vi "GoT (SubVI).vi"(0 "Error In 3":errorcluster, 1 "Error In 9":errorcluster, 5 "error in (no error)":errorcluster) -> (6 "Selected Octave 3":i32[](array[numeric]), 8 "Number_of_elements 9":dbl, 9 "Array 2":i32[](array[numeric]), 10 "Number_of_elements 3":dbl, 11 "Notes 2":i32[](array[numeric]), 12 "Status 3":i32[](array[numeric]), 13 "Time 2":dbl[](array[numeric]), 14 "Array 3":dbl[](array[numeric]), 15 "Error Out 3":errorcluster, 16 "Array":i32[](array[numeric]), 17 "Error Out 9":errorcluster, 18 "Number_of_elements 4":dbl, 19 "error out":errorcluster)   [LabVIEW 2016]
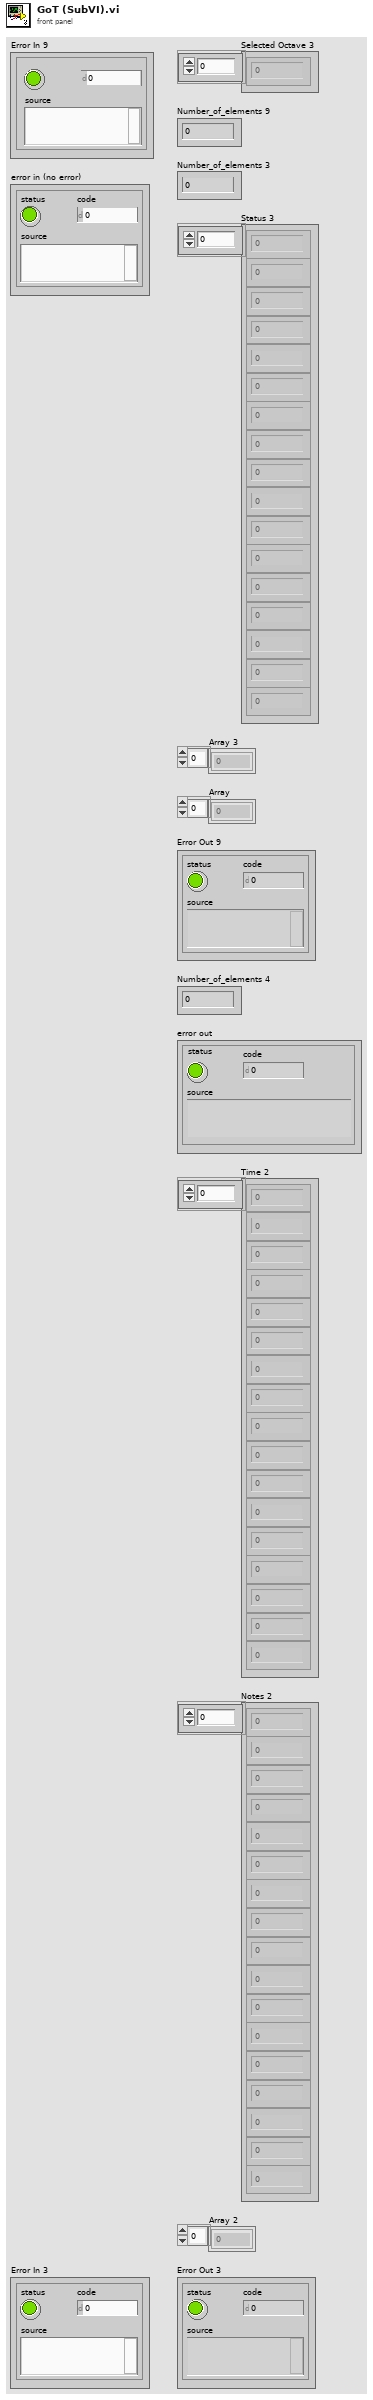
[diagram p1: front panel]
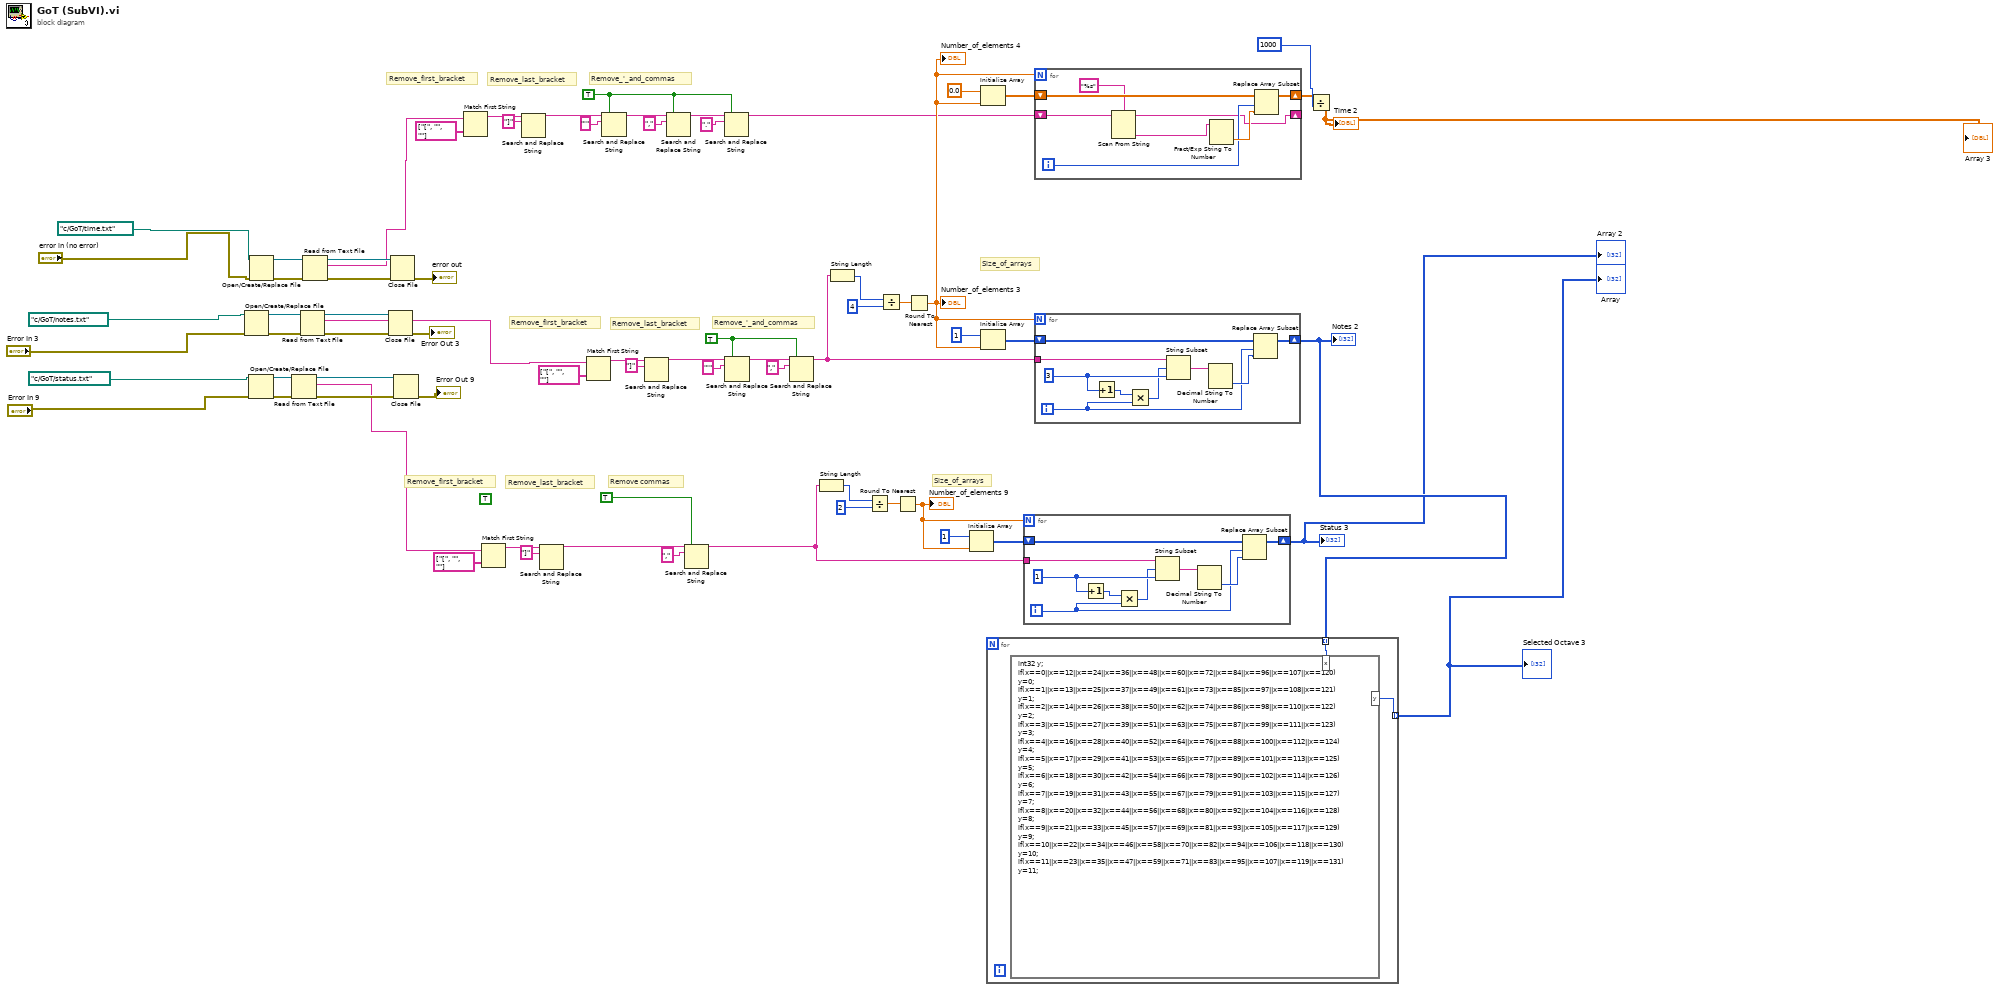
[diagram p0: block diagram]
diagram:
  (unwired) TRUE ("replace all? (F)")
  w13 = TRUE ("replace all? (F)")
  w27 = TRUE ("replace all? (F)")
  # "Size_of_arrays"
  # "Remove commas"
  # "Remove_last_bracket"
  # "Remove_first_bracket"
  # "Remove_'_and_commas"
  # "Remove_last_bracket"
  # "Remove_first_bracket"
  # "Size_of_arrays"
  # "Remove_'_and_commas"
  # "Remove_last_bracket"
  # "Remove_first_bracket"
  n1 = Open/Create/Replace File(file path (use dialog)=path "c:/GoT/notes.txt", error in="Error In 3") -> (refnum out=w65:refnum<file>, error out=w66:errorcluster)  [unwired: 4 in, 1 out]
  n2 = Open/Create/Replace File(file path (use dialog)=path "c:/GoT/status.txt", error in="Error In 9") -> (refnum out=w68:refnum<file>, error out=w67:errorcluster)  [unwired: 4 in, 1 out]
  n3 = Open/Create/Replace File(file path (use dialog)=path "c:/GoT/time.txt", error in="error in (no error)") -> (refnum out=w58:refnum<file>, error out=w57:errorcluster)  [unwired: 4 in, 1 out]
  n4 = Read from Text File(file (use dialog)=w68, error in=w67) -> (refnum out=w70:refnum<file>, text=w52:string, error out=w69:errorcluster)  [unwired: 2 in, 1 out]
  n5 = Read from Text File(file (use dialog)=w65, error in=w66) -> (refnum out=w62:refnum<file>, text=w33:string, error out=w63:errorcluster)  [unwired: 2 in, 1 out]
  n6 = Read from Text File(file (use dialog)=w58, error in=w57) -> (refnum out=w61:refnum<file>, text=w31:string, error out=w60:errorcluster)  [unwired: 2 in, 1 out]
  n7 = Close File(refnum=w62, error in=w63) -> (error out=→"Error Out 3":errorcluster)  [unwired: 1 out]
  n8 = Close File(refnum=w61, error in=w60) -> (error out=→"error out":errorcluster)  [unwired: 1 out]
  n9 = Close File(refnum=w70, error in=w69) -> (error out=→"Error Out 9":errorcluster)  [unwired: 1 out]
  n10 = Match First String(2:string[] ["[", "", ""] ("string array"), 3:w31) -> (1:w2:string)  [unwired: 1 out]
  n11 = Match First String(2:string[] ["[", "", ""] ("string array"), 3:w52) -> (1:w40:string)  [unwired: 1 out]
  n12 = Search and Replace String(input string=w2, search string="]") -> (result string=w4:string)  [unwired: 6 in, 3 out]
  n13 = Search and Replace String(input string=w40, search string="]") -> (result string=w42:string)  [unwired: 6 in, 3 out]
  n14 = Match First String(2:string[] ["[", "", ""] ("string array"), 3:w33) -> (1:w22:string)  [unwired: 1 out]
  n15 = Search and Replace String(replace all?=w27, input string=w4, search string="'") -> (result string=w7:string)  [unwired: 5 in, 3 out]
  n16 = Search and Replace String(input string=w22, search string="]") -> (result string=w20:string)  [unwired: 6 in, 3 out]
  n17 = Search and Replace String(replace all?=w27, input string=w7, search string=",") -> (result string=w24:string)  [unwired: 5 in, 3 out]
  n18 = Search and Replace String(replace all?=TRUE ("replace all? (F)"), input string=w42, search string=",") -> (result string=w49:string)  [unwired: 5 in, 3 out]
  n19 = Search and Replace String(replace all?=w27, input string=w24, search string=".") -> (result string=w25:string)  [unwired: 5 in, 3 out]
  n20 = Search and Replace String(replace all?=w13, input string=w20, search string="'") -> (result string=w17:string)  [unwired: 5 in, 3 out]
  n21 = Search and Replace String(replace all?=w13, input string=w17, search string=",") -> (result string=w12:string)  [unwired: 5 in, 3 out]
  n22 = String Length(string=w49) -> (length=w47:i32)
  n23 = String Length(string=w12) -> (length=w16:i32)
  n24 = Divide(x=w47, y=2) -> (x/y=w45:dbl)
  n25 = Divide(x=w16, y=4) -> (x/y=w14:dbl)
  n26 = Round To Nearest(number=w45) -> (nearest integer value=w48:dbl)
  "Number_of_elements 9" <- w48
  n27 = Round To Nearest(number=w14) -> (nearest integer value=w34:dbl)
  "Number_of_elements 4" <- w34
  "Number_of_elements 3" <- w34
  n28 = Initialize Array(1 ("Number_of_elements"), w48) -> (w43:i32[])
  n29 = Initialize Array(0.0 ("Number_of_elements"), w34) -> (w9:dbl[])
  n30 = Initialize Array(1 ("Number_of_elements"), w34) -> (w10:i32[])
  n31 = for {
    N: w48 -> [_]
    tunnel: w49 -> [w80]
    shift-right: [w72] -> w54
    shift-left: w43 -> [w75]
    i -> [w73]
    w79 = 1 ("length (rest)")
    n32 = Increment(x=w79) -> (x+1=w78:i32)
    n33 = Multiply(x=w78, y=w73) -> (x*y=w77:i32)
    n34 = String Subset(string=w80, offset (0)=w77, length (rest)=w79) -> (substring=w76:string)
    n35 = Decimal String To Number(string=w76) -> (number=w74:i32)  [unwired: 2 in, 1 out]
    n36 = Replace Array Subset(array=w75, new element=w74, index=w73) -> (w72:i32[])
  }
  "Status 3" <- w54
  "Array 2" <- w54
  n37 = for {
    N: w34 -> [_]
    tunnel: w12 -> [w89]
    shift-right: [w81] -> w55
    shift-left: w10 -> [w84]
    i -> [w82]
    w88 = 3 ("length (rest)")
    n38 = Increment(x=w88) -> (x+1=w87:i32)
    n39 = Multiply(x=w87, y=w82) -> (x*y=w86:i32)
    n40 = String Subset(string=w89, offset (0)=w86, length (rest)=w88) -> (substring=w85:string)
    n41 = Decimal String To Number(string=w85) -> (number=w83:i32)  [unwired: 2 in, 1 out]
    n42 = Replace Array Subset(array=w84, new element=w83, index=w82) -> (w81:i32[])
  }
  "Notes 2" <- w55
  n43 = for {
    tunnel: w55 -> [w91] mode=indexing
    tunnel: [w90] -> w56 mode=indexing
    n44 = formula code="int32 y;\nif(x==0||x==12||x==24||x==36||x==48||x==60||x==72||x==84||x==96||x==107||x==120)\ny=0;\nif(x==1||x==13||x==25||x==37||x==49||x==61||x==73||x==85||x==97||x==108||x==121)\ny=1;\nif(x==2||x==14||x==26||x==38||x==50||x==62||x==74||x==86||x==98||x==110||x==122)\ny=2;\nif(x==3||x==15||x==27||x==39||x==51||x==63||x==75||x==87||x==99||x==111||x==123)\ny=3;\nif(x==4||x==16||x==28||x==40||x==52||x==64||x==76||x==88||x==100||x==112||x==124)\ny=4;\nif(x==5||x==17||x==29||x==41||x==53||x==65||x==77||x==89||x==101||x==113||x==125)\ny=5;\nif(x==6||x==18||x==30||x==42||x==54||x==66||x==78||x==90||x==102||x==114||x==126)\ny=6;\nif(x==7||x==19||x==31||x==43||x==55||x==67||x==79||x==91||x==103||x==115||x==127)\ny=7;\nif(x==8||x==20||x==32||x==44||x==56||x==68||x==80||x==92||x==104||x==116||x==128)\ny=8;\nif(x==9||x==21||x==33||x==45||x==57||x==69||x==81||x==93||x==105||x==117||x==129)\ny=9;\nif(x==10||x==22||x==34||x==46||x==58||x==70||x==82||x==94||x==106||x==118||x==130)\ny=10;\nif(x==11||x==23||x==35||x==47||x==59||x==71||x==83||x==95||x==107||x==119||x==131)\ny=11;"("x"=w91) -> ("y"=w90:i32)
  }
  "Selected Octave 3" <- w56
  "Array" <- w56
  n45 = for {
    N: w34 -> [_]
    shift-right: [w96] -> w28
    shift-left: w9 -> [w99]
    shift-right: [w92] -> _
    shift-left: w25 -> [w94]
    i -> [w97]
    n46 = Scan From String(format string="%s", input string=w94) -> (remaining string=w92:string, output 1=w93:string)  [unwired: 3 in, 2 out]
    n47 = Fract/Exp String To Number(string=w93) -> (number=w98:dbl)  [unwired: 3 in, 1 out]
    n48 = Replace Array Subset(array=w99, new element=w98, index=w97) -> (w96:dbl[])
  }
  n49 = Divide(x=w28, y=1000 ("length (rest)")) -> (x/y=→"Time 2" →"Array 3":dbl[])
